vi "SetIcon.vi"(8 "error in (no error)":errorcluster, 9 "Icon":T1, 10 "Tag Name":string, 11 "ResultTree in":refnum<class "ResultTree.lvclass">) -> (0 "error out":errorcluster, 3 "ResultTree out":refnum<class "ResultTree.lvclass">)   [LabVIEW 2017, in "ResultTree.lvclass"]
doc: "Sets the icon."
uses:
  ResultTree.lvclass
  Icon.ctl
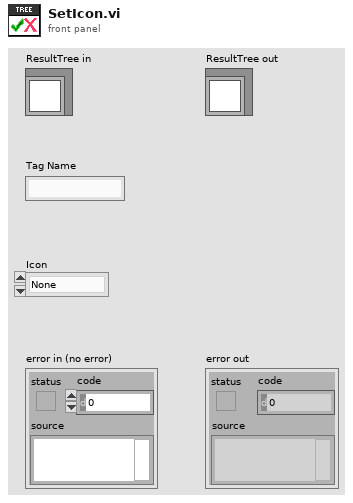
[diagram p1: front panel]
types:
  T1 = typedef "ResultTree.lvclass/Icon.ctl" = enum16{"None", "Passed", "Failed", "Error"}
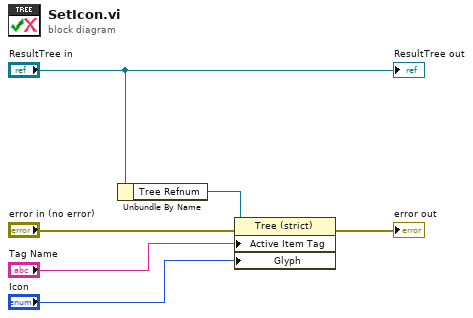
[diagram p0: block diagram]
diagram:
  n1 = Unbundle By Name("ResultTree in") -> ("Tree Refnum"=w3:refnum<vi>)
  n2 = property class="Tree (strict)"(reference=w3, error in="error in (no error)", "Active Item Tag"="Tag Name", "Glyph"="Icon") -> (error out=→"error out":errorcluster)  [unwired: 1 out]
  "ResultTree out" <- "ResultTree in"
